vi "MT2Hours.vi"() -> ()   [LabVIEW 2012]
uses:
  <vilib>/addons/database/Auxilliary.llb/DB Tools Cursor Type.ctl
  <vilib>/Utility/NIReport.llb/NI_report.lvclass
  <vilib>/addons/database/Connection.llb/DB Tools Open Connec (Path).vi
  <vilib>/addons/database/Connection.llb/Conn Execute.vi
  <vilib>/addons/database/Recordset.llb/Rec Fetch Recordset Data (R).vi
  <vilib>/addons/database/Recordset.llb/Rec Destroy - Connection.vi
  <vilib>/addons/database/_DB Variant To Data/Database Variant To Data.xnode
  <vilib>/addons/database/NI_Database_API.lvlib
  <vilib>/Utility/NIReport.llb/Excel/NI_Excel.lvclass
  <vilib>/Utility/SMTP/NI_SMTPEmail.lvlib
panel:
  out "error out 3":errorcluster
  in  "MIME content-type (application/octet-stream)":string="application/octet-stream"
  out "error out 2":errorcluster
  in  "?":cluster{"start row":i32, "start column":i32}
  out "error out":errorcluster
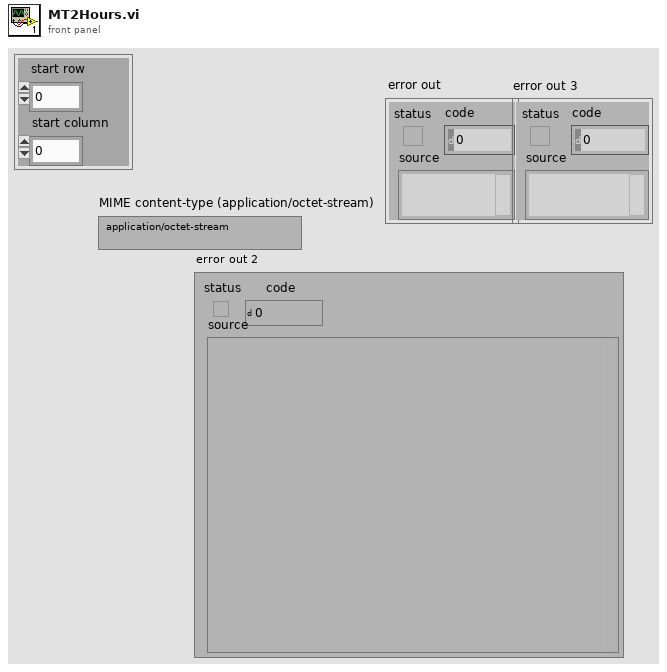
[diagram p1: front panel]
types:
  T1 = enum16{"Standard Report", "HTML", "Word", "Excel"}
  T2 = typedef "NI_Database_API.lvlib/Conn ObjectReference.ctl" = refnum<k1>
  T3 = typedef "NI_Database_API.lvlib/DB Tools Cursor Type.ctl" = enum16{"forward-only", "keyset", "dynamic", "static"}
  T4 = typedef "NI_Database_API.lvlib/Rec ObjectReference.ctl" = refnum<k1>
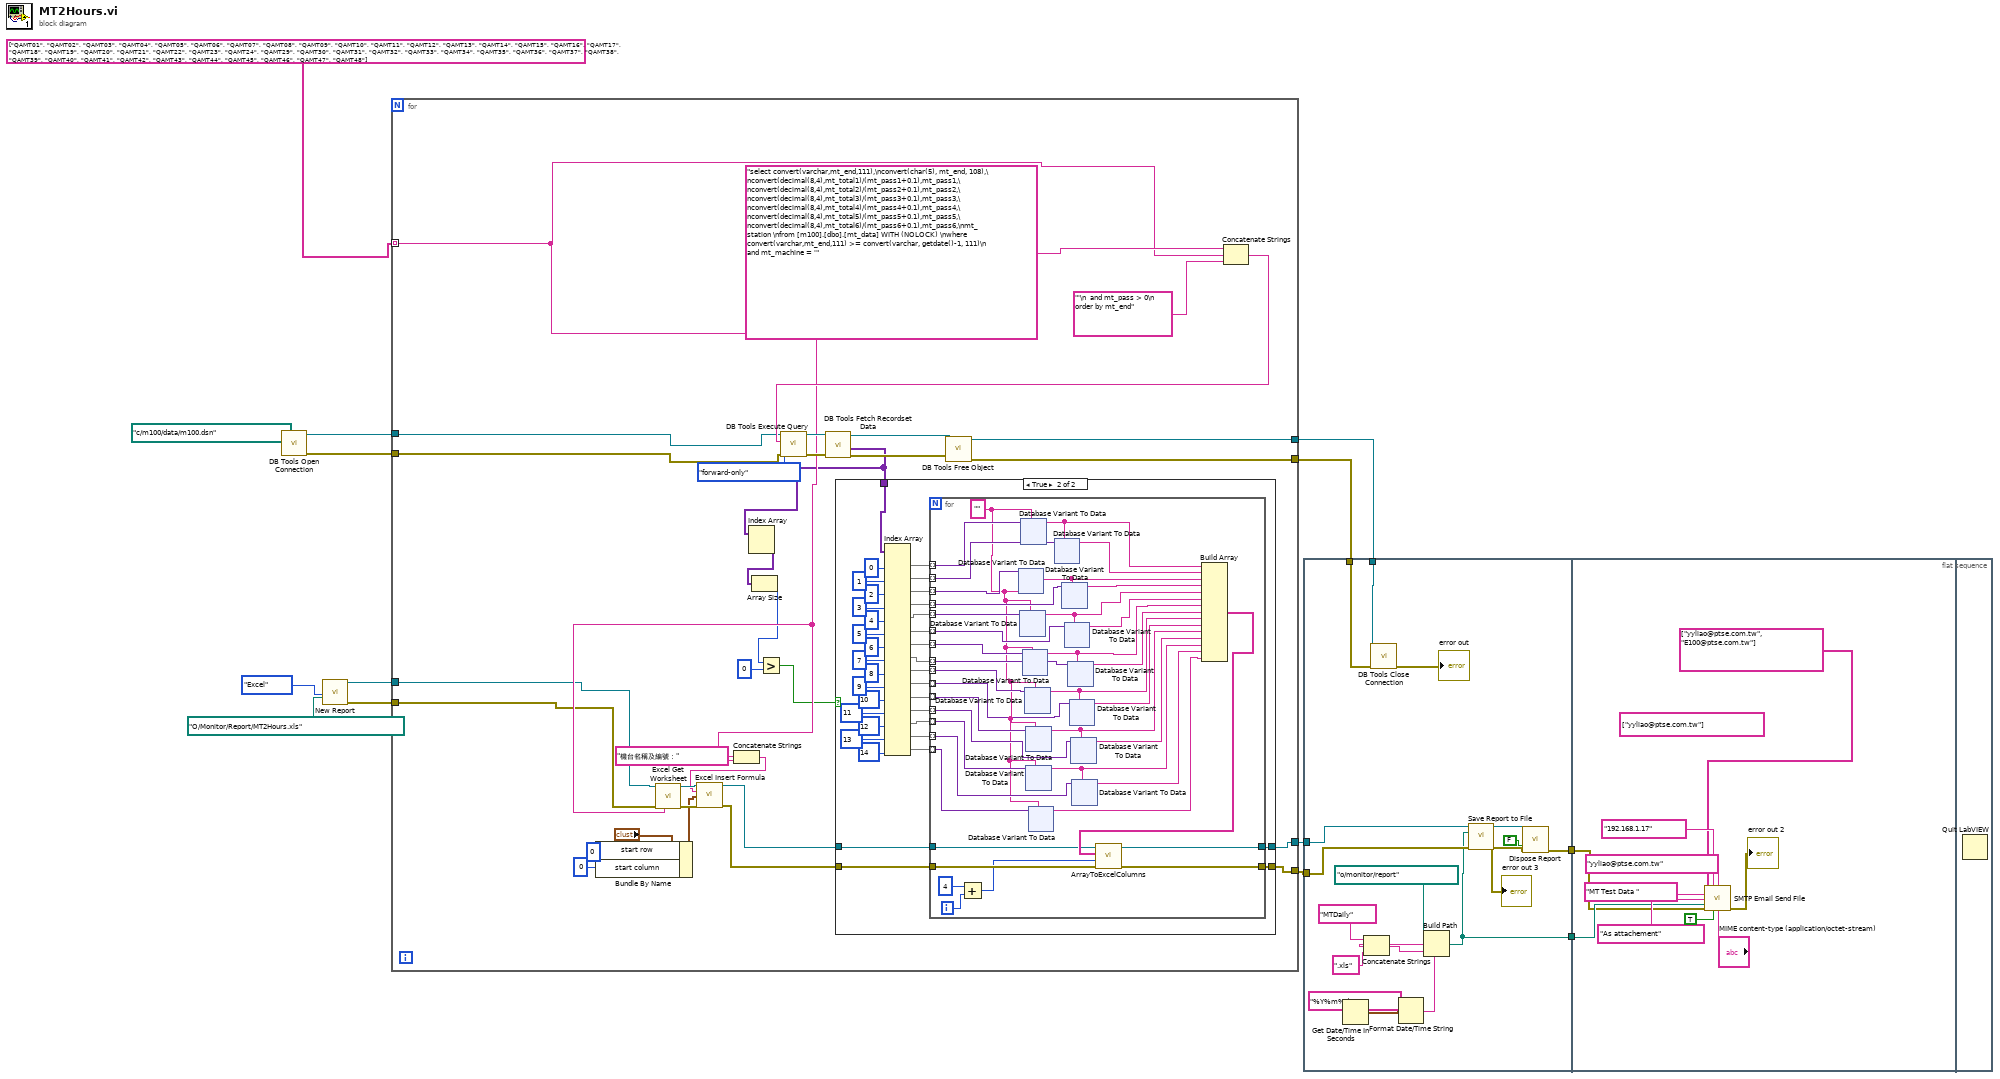
[diagram p0: block diagram]
diagram:
  n1 = call-poly <vilib>:"DB Tools Open Connection.vi"("connection information"=path "c:/m100/data/m100.dsn") -> ("error out"=w6:errorcluster, "connection reference"=w7:T2)  [unwired: 7 in]
  n2 = call <vilib>:"New Report.vi"("report type"=T1."Excel" ("Report Type"), "template (empty)"=path "O:/Monitor/Report/MT2Hours.xls") -> ("report out"=w10:refnum<class "NI_report.lvclass">, "error out"=w9:errorcluster)  [unwired: 12 in]
  n3 = for {
    tunnel: [w28] -> w14
    tunnel: [w27] -> w13
    tunnel: string[] ["QAMT01", "QAMT02", "QAMT03", "QAMT04", "QAMT05", "QAMT06", "QAMT07", "QAMT08", "QAMT09", "QAMT10", "QAMT11", "QAMT12", "QAMT13", "QAMT14", "QAMT15", "QAMT16", "QAMT17", "QAMT18", "QAMT19", "QAMT20", "QAMT21", "QAMT22", "QAMT23", "QAMT24", "QAMT29", "QAMT30", "QAMT31", "QAMT32", "QAMT33", "QAMT34", "QAMT35", "QAMT36", "QAMT37", "QAMT38", "QAMT39", "QAMT40", "QAMT41", "QAMT42", "QAMT43", "QAMT44", "QAMT45", "QAMT46", "QAMT47", "QAMT48"] ("Array") -> [w26] mode=indexing
    tunnel: w10 -> [w25]
    tunnel: w9 -> [w24]
    tunnel: w7 -> [w23]
    tunnel: w6 -> [w22]
    tunnel: [w21] -> w4
    tunnel: [w20] -> w3
    n4 = Bundle By Name(cluster="?", "start row"=0, "start column"=0) -> (w33:cluster{"start row":i32, "start column":i32})
    n5 = call <vilib>:"Excel Get Worksheet.vi"("report in"=w25, "error in (no error)"=w24, "name (\"\")"=w26) -> ("report out"=w38:refnum<class "NI_report.lvclass">, "error out"=w37:errorcluster)  [unwired: 11 in]
    n6 = Concatenate Strings("機台名稱及編號：" ("formula"), w26) -> (w30:string)
    n7 = call <vilib>:"Excel Insert Formula.vi"("report in"=w38, "formula"=w30, "start (0, 0)"=w33, "error in (no error)"=w37) -> ("report out"=w32:refnum<class "NI_report.lvclass">, "error out"=w31:errorcluster)  [unwired: 10 in]
    n8 = Concatenate Strings("select convert(varchar,mt_end,111),\nconvert(char(5), mt_end, 108),\nconvert(decimal(8,4),mt_total1)/(mt_pass1+0.1),mt_pass1,\nconvert(decimal(8,4),mt_total2)/(mt_pass2+0.1),mt_pass2,\nconvert(decimal(8,4),mt_total3)/(mt_pass3+0.1),mt_pass3,\nconvert(decimal(8,4),mt_total4)/(mt_pass4+0.1),mt_pass4,\nconvert(decimal(8,4),mt_total5)/(mt_pass5+0.1),mt_pass5,\nconvert(decimal(8,4),mt_total6)/(mt_pass6+0.1),mt_pass6,\nmt_station \nfrom [m100].[dbo].[mt_data] WITH (NOLOCK) \nwhere convert(varchar,mt_end,111) >= convert(varchar, getdate()-1, 111)\n  and mt_machine = '" ("SQL query"), w26, "'\n  and mt_pass > 0\n  order by mt_end" ("SQL query")) -> (w39:string)
    n9 = call-poly <vilib>:"DB Tools Execute Query.vi"("error in (no error)"=w22, "cursor type"=DB_Tools_Cursor_Type."forward-only", "SQL query"=w39, "connection reference"=w23) -> ("error out"=w46:errorcluster, "recordset reference"=w45:T4)  [unwired: 4 in]
    n10 = call-poly <vilib>:"DB Tools Fetch Recordset Data.vi"("error in (no error)"=w46, "recordset reference"=w45) -> ("error out"=w43:errorcluster, "recordset data"=w19:variant[][], "recordset reference out"=w44:T4)  [unwired: 3 in]
    n11 = Index Array(array=w19) -> (element=w18:variant[])  [unwired: 2 in]
    n12 = Array Size(array=w18) -> (size(s)=w17:i32)
    n13 = Greater?(x=w17, y=0) -> (0:w15:bool)
    n14 = case shown="True" w15 {
      tunnel: w19 -> [_ w83]
      tunnel: w32 -> [w48 w54]
      tunnel: w31 -> [w47 w53]
      tunnel: [w48 w52] -> w28
      tunnel: [w47 w51] -> w27
      frame False {
      }
      frame True {
        n15 = Index Array(array=w83, index (col) #1=0 ("disabled index (col)"), index (col) #2=1 ("index (col)"), index (col) #3=2 ("index (col)"), index (col) #4=3 ("index (col)"), index (col) #5=4 ("index (col)"), index (col) #6=5 ("index (col)"), index (col) #7=6 ("index (col)"), index (col) #8=7 ("index (col)"), index (col) #9=8 ("index (col)"), index (col) #10=9 ("index (col)"), index (col) #11=10 ("index (col)"), index (col) #12=11 ("index (col)"), index (col) #13=12 ("index (col)"), index (col) #14=13 ("index (col)"), index (col) #15=14 ("index (col)")) -> (element #1=w80:variant[], element #2=w79:variant[], element #3=w78:variant[], element #4=w67:variant[], element #5=w66:variant[], element #6=w65:variant[], element #7=w64:variant[], element #8=w63:variant[], element #9=w62:variant[], element #10=w61:variant[], element #11=w60:variant[], element #12=w59:variant[], element #13=w56:variant[], element #14=w55:variant[], element #15=w49:variant[])  [unwired: 15 in]
        n16 = for {
          tunnel: w80 -> [w122] mode=indexing
          tunnel: w79 -> [w121] mode=indexing
          tunnel: w78 -> [w120] mode=indexing
          tunnel: w67 -> [w118] mode=indexing
          tunnel: w66 -> [w114] mode=indexing
          tunnel: w65 -> [w112] mode=indexing
          tunnel: w64 -> [w110] mode=indexing
          tunnel: w63 -> [w107] mode=indexing
          tunnel: w62 -> [w106] mode=indexing
          tunnel: w61 -> [w105] mode=indexing
          tunnel: w60 -> [w102] mode=indexing
          tunnel: w59 -> [w101] mode=indexing
          tunnel: w56 -> [w98] mode=indexing
          tunnel: w55 -> [w97] mode=indexing
          tunnel: w54 -> [w93]
          tunnel: w53 -> [w92]
          tunnel: [w88] -> w52
          tunnel: [w87] -> w51
          tunnel: w49 -> [w86] mode=indexing
          i -> [w91]
          w85 = ""
          n17 = Add(x=4, y=w91) -> (x+y=w89:i32)
          n18 = xnode "Database Variant To Data"("database variant"=w120, "type"=w85) -> ("data"=w116:string)  [unwired: 1 in, 1 out]
          n19 = xnode "Database Variant To Data"("database variant"=w114, "type"=w85) -> ("data"=w113:string)  [unwired: 1 in, 1 out]
          n20 = xnode "Database Variant To Data"("database variant"=w122, "type"=w85) -> ("data"=w117:string)  [unwired: 1 in, 1 out]
          n21 = xnode "Database Variant To Data"("database variant"=w110, "type"=w85) -> ("data"=w109:string)  [unwired: 1 in, 1 out]
          n22 = xnode "Database Variant To Data"("database variant"=w106, "type"=w85) -> ("data"=w104:string)  [unwired: 1 in, 1 out]
          n23 = xnode "Database Variant To Data"("database variant"=w102, "type"=w85) -> ("data"=w100:string)  [unwired: 1 in, 1 out]
          n24 = xnode "Database Variant To Data"("database variant"=w98, "type"=w85) -> ("data"=w96:string)  [unwired: 1 in, 1 out]
          n25 = xnode "Database Variant To Data"("database variant"=w86, "type"=w85) -> ("data"=w84:string)  [unwired: 1 in, 1 out]
          n26 = xnode "Database Variant To Data"("database variant"=w121, "type"=w117) -> ("data"=w119:string)  [unwired: 1 in, 1 out]
          n27 = xnode "Database Variant To Data"("database variant"=w118, "type"=w116) -> ("data"=w115:string)  [unwired: 1 in, 1 out]
          n28 = xnode "Database Variant To Data"("database variant"=w112, "type"=w113) -> ("data"=w111:string)  [unwired: 1 in, 1 out]
          n29 = xnode "Database Variant To Data"("database variant"=w107, "type"=w109) -> ("data"=w108:string)  [unwired: 1 in, 1 out]
          n30 = xnode "Database Variant To Data"("database variant"=w105, "type"=w104) -> ("data"=w103:string)  [unwired: 1 in, 1 out]
          n31 = xnode "Database Variant To Data"("database variant"=w101, "type"=w100) -> ("data"=w99:string)  [unwired: 1 in, 1 out]
          n32 = xnode "Database Variant To Data"("database variant"=w97, "type"=w96) -> ("data"=w95:string)  [unwired: 1 in, 1 out]
          n33 = Build Array(w117, w119, w116, w115, w113, w111, w109, w108, w104, w103, w100, w99, w96, w95, w84) -> (w94:string[])
          n34 = call "ArrayToExcelColumns.vi"("error in (no error)"=w92, "start row"=w89, "ArrayData"=w94, "report in"=w93) -> ("error in (no error) 2"=w87:errorcluster, "report in 2"=w88:refnum<class "NI_report.lvclass">)  [unwired: 6 in]
        }
      }
    }
    n35 = call-poly <vilib>:"DB Tools Free Object.vi"("error in (no error)"=w43, "recordset reference"=w44) -> ("error out"=w20:errorcluster, "connection reference"=w21:T2)  [unwired: 8 in]
  }
  n36 = flat-sequence {
    tunnel: w14 -> [w615]
    tunnel: w13 -> [w614]
    tunnel: w4 -> [w605]
    tunnel: w3 -> [w604]
    tunnel: [w608] -> w2
    tunnel: [w607] -> w1
    tunnel: w2 -> [w621]
    tunnel: w1 -> [w622]
    frame #0 {
      n37 = Get Date/Time In Seconds() -> (seconds since 1Jan1904=w611:timestamp)
      n38 = call <vilib>:"DB Tools Close Connection.vi"("error in (no error)"=w604, "connection reference"=w605) -> ("error out"=→"error out":errorcluster)  [unwired: 5 in]
      n39 = Format Date/Time String(time format string (%c)="%Y%m%d%H", seconds (now)=w611) -> (date/time string=w609:string)  [unwired: 1 in]
      n40 = Concatenate Strings("MTDaily" ("string"), w609, ".xls" ("string")) -> (w616:string)
      n41 = Build Path(base path=path "o:/monitor/report", name or relative path=w616) -> (appended path=w607:path)
      n42 = call-dynamic "Save Report to File.vi"("report in"=w615, "report file path"=w607, "error in (no error)"=w614) -> ("report out"=w618:refnum<class "NI_report.lvclass">, "error out"=w617:errorcluster)  [unwired: 11 in]
      "error out 3" <- w617
      n43 = call-dynamic "Dispose Report.vi"("report in"=w618, "save changes? (F)"=FALSE, "error in (no error)"=w617) -> ("error out"=w608:errorcluster)  [unwired: 12 in]
    }
    frame #1 {
      (unwired) string[] ["yyliao@ptse.com.tw"] ("recipients")
      n44 = call <vilib>:"SMTP Email Send File.vi"("recipients"=string[] ["yyliao@ptse.com.tw", "E100@ptse.com.tw"], "mail server"="192.168.1.17", "return address"="yyliao@ptse.com.tw", "subject ([No Subject])"="MT Test Data ", "message"="As attachement", "file path"=w622, "error in (no error)"=w621, "binary? (F)"=TRUE, "MIME content-type (application/octet-stream)"="MIME content-type (application/octet-stream)") -> ("error out"=→"error out 2":errorcluster)  [unwired: 5 in, 1 out]
    }
    frame #2 {
      n45 = Quit LabVIEW() -> ()  [unwired: 1 in]
    }
  }
